vi "TTA_MATLAB_SetRFICsWithWhomTalking.vi"(0 "Panel Array":i32[](array[numeric])=[1, 2], 5 "RFIC Array":i32[](array[numeric])=[1, 2, 3, 4, 5, 6, 7, 8, 9, 10, 11, 12, 13, 14, 15, 16, 17, 18, 19, 20, 21, 22, 23, 24], 11 "error in":errorcluster) -> (15 "error out":errorcluster)   [LabVIEW 2016]
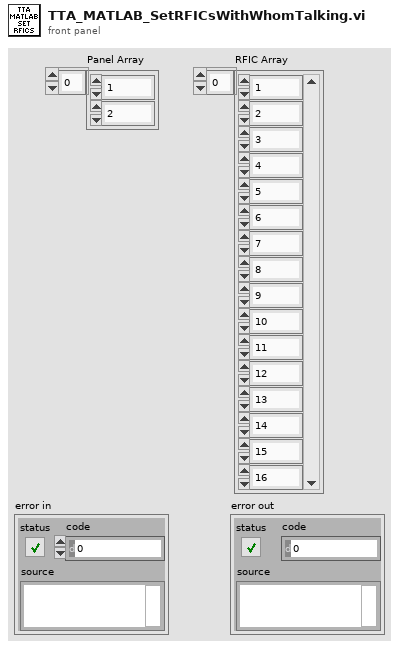
[diagram p1: front panel]
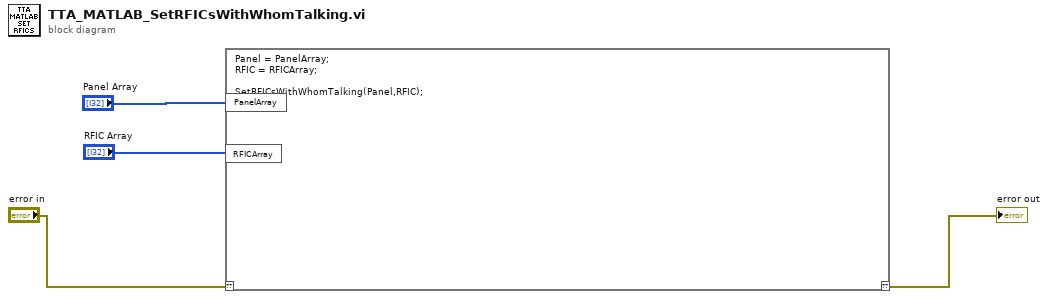
[diagram p0: block diagram]
diagram:
  n1 = script code="Panel = PanelArray;\nRFIC = RFICArray;\n\nSetRFICsWithWhomTalking(Panel,RFIC);"("??"="error in", "PanelArray"="Panel Array", "RFICArray"="RFIC Array") -> ("??"=→"error out":errorcluster)
